vi "Init FIU page.vi"(7 "Card Position":refnum<vi>, 8 "error in (no error)":errorcluster, 9 "Description":refnum<vi>, 10 "Name":refnum<vi>, 11 "Node Ptr":T2 format="%.0x") -> (0 "error out":errorcluster, 2 "Fault States":T1[](array[typedef]), 3 "Node Ptr out":T2 format="%.0x")   [LabVIEW 2014, in "SLSC configuration System Explorer.lvlib"]
uses:
  SLSC configuration System Explorer.lvlib
  <vilib>/NI Veristand/Custom Device API/Custom Device Item Ref.ctl
  Example/FIU Board/Fault State.ctl
  Type Defs/Card Position.ctl
  Example/SPI Utility/Slot #.ctl
  Shared/Constants.vi
  <vilib>/NI Veristand/Custom Device API/Get Item Property (U16).vi
  <vilib>/NI Veristand/Custom Device API/Custom Device API.lvlib
  Shared/SLSC configuration Shared.lvlib
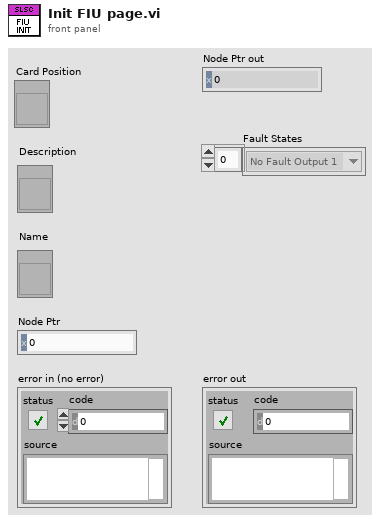
[diagram p1: front panel]
types:
  T1 = typedef "SLSC configuration Shared.lvlib/Fault State.ctl" = enum8{"No Fault Output 1", "Open Circuit 100 Hz", "Ground 100 Hz", "Open Circuit", "Ground", "Fail Rail 1", "Fail Rail 2", "No Fault Output 2"}
  T2 = typedef "Custom Device API.lvlib/Custom Device Item Ref.ctl" = u64
  T3 = typedef "SLSC configuration Shared.lvlib/Card Position.ctl" = cluster{"Rack #":u8, "Slot #":T4}
  T4 = typedef "SLSC configuration Shared.lvlib/Slot #.ctl" = u8
  T5 = typedef "Custom Device API.lvlib/Custom Device Item Info.ctl" = cluster{"Name":string, "Is Channel":bool, "GUID":string, "Is Waveform":bool}
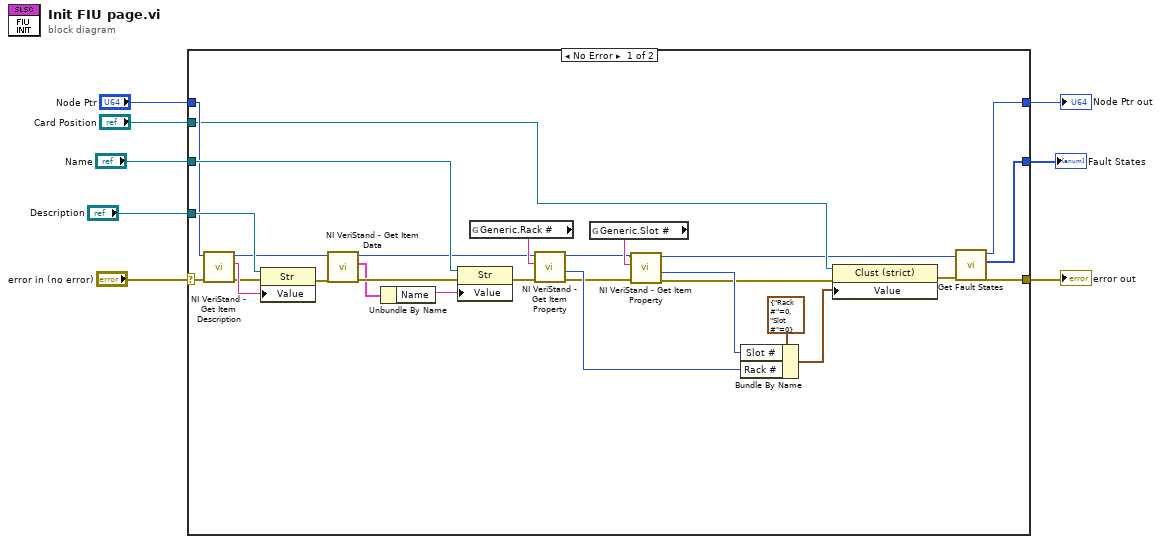
[diagram p0: block diagram]
diagram:
  n1 = case shown="No Error" "error in (no error)" {
    selector: "error in (no error)" -> [w23 w38]
    tunnel: "Name" -> [w36 _]
    tunnel: "Description" -> [w32 _]
    tunnel: [w28 w38] -> w6
    tunnel: "Node Ptr" -> [w27 w37]
    tunnel: "Card Position" -> [w21 _]
    tunnel: [w10 _] -> w1
    tunnel: [w9 w37] -> w2
    frame No Error {
      n2 = call <vilib>:"NI VeriStand - Get Item Description.vi"("error in (no error)"=w23, "Item Ref in"=w27) -> ("error out"=w31:errorcluster, "Description"=w33:string, "Item Ref out"=w29:T2)  [unwired: 7 out]
      n3 = property class="Str"(reference=w32, error in=w31, "Value"=w33) -> (error out=w34:errorcluster)  [unwired: 1 out]
      n4 = call <vilib>:"NI VeriStand - Get Item Data.vi"("error in (no error)"=w34, "Item Ref in"=w29) -> ("error out"=w35:errorcluster, "Item Info"=w30:T5, "Item Ref out"=w24:T2)  [unwired: 7 out]
      n5 = Unbundle By Name(w30) -> ("Name"=w20:string)
      n6 = property class="Str"(reference=w36, error in=w35, "Value"=w20) -> (error out=w25:errorcluster)  [unwired: 1 out]
      n7 = global read "Constants.vi" "Generic.Rack #"() -> (w26:string)
      n8 = call-poly <vilib>:"NI VeriStand - Get Item Property.vi"("error in (no error)"=w25, "Property Name"=w26, "Item Ref in"=w24) -> ("error out"=w16:errorcluster, "Value"=w18:u16, "Item Ref out"=w14:T2)  [unwired: 5 in, 1 out]
      n9 = global read "Constants.vi" "Generic.Slot #"() -> (w15:string)
      n10 = call-poly <vilib>:"NI VeriStand - Get Item Property.vi"("error in (no error)"=w16, "Property Name"=w15, "Item Ref in"=w14) -> ("error out"=w11:errorcluster, "Value"=w12:u16, "Item Ref out"=w13:T2)  [unwired: 5 in, 1 out]
      n11 = Bundle By Name(cluster=T3 {"Rack #"=0, "Slot #"=0} ("Card Position"), "Slot #"=w12, "Rack #"=w18) -> (w17:T3)
      n12 = property class="Clust (strict)"(reference=w21, error in=w11, "Value"=w17) -> (error out=w22:errorcluster)  [unwired: 1 out]
      n13 = call "Get Fault States.vi"("error in (no error)"=w22, "FIU Board Ref in"=w13) -> ("error out"=w28:errorcluster, "Fault States"=w10:T1[], "FIU Board Ref out"=w9:T2)  [unwired: 6 in, 1 out]
    }
    frame Error {
    }
  }
  "Node Ptr out" <- w2
  "error out" <- w6
  "Fault States" <- w1
